vi "Drive_Utils_setRobotState.vi"(8 "error in (no error)":errorcluster, 11 "Robot State":T1) -> (0 "error out":errorcluster)   [LabVIEW 2009, in "Drive.lvlib" / "Drive_Utils.lvlib"]
uses:
  Drive_Utils.lvlib
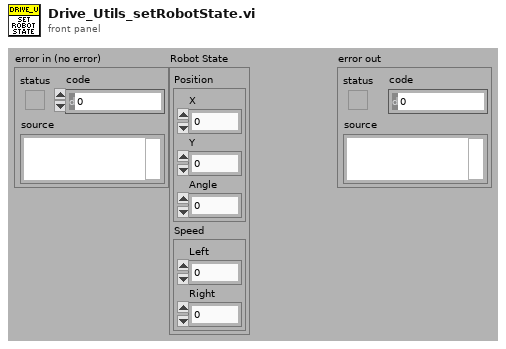
[diagram p1: front panel]
types:
  T1 = cluster{"Position":cluster{"X":dbl, "Y":dbl, "Angle":dbl}, "Speed":cluster{"Left":dbl, "Right":dbl}}
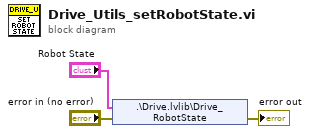
[diagram p0: block diagram]
diagram:
  n1 = shared-variable ".\\Drive.lvlib\\Drive_RobotState"("Robot State", error in="error in (no error)") -> (error out=→"error out":errorcluster)
